vi "ControlMain.vi"() -> ()   [LabVIEW 2022 SP3]
panel:
  out "data out":string
  in  "stop":bool
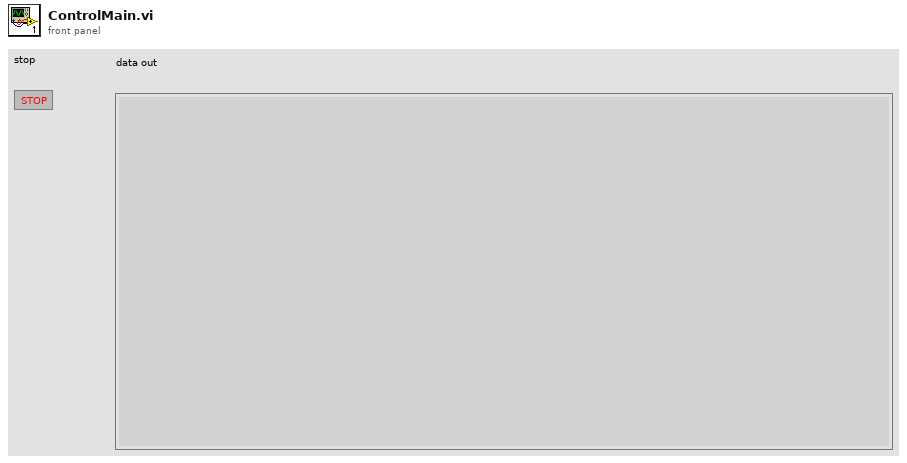
[diagram p1: front panel]
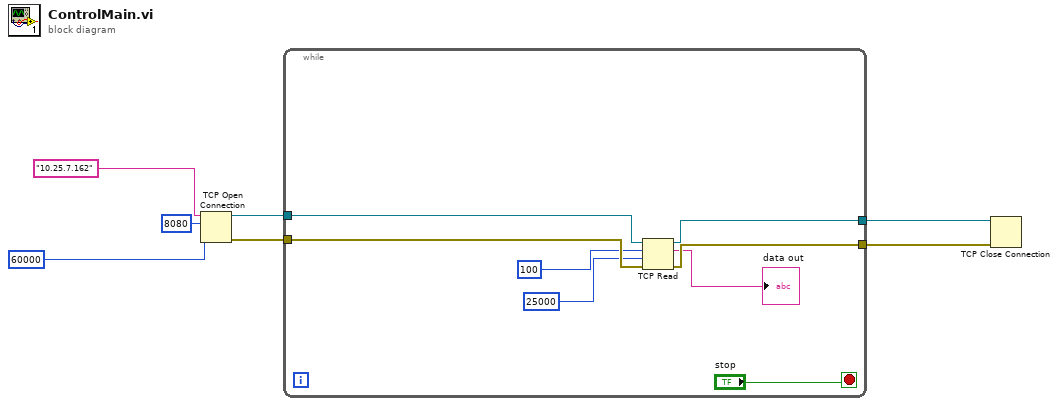
[diagram p0: block diagram]
diagram:
  n1 = TCP Open Connection(address="10.25.7.162", remote port or service name=u16 8080, timeout ms (60000)=60000) -> (connection ID=w3:refnum<k5>, error out=w4:errorcluster)  [unwired: 2 in]
  n2 = while {
    tunnel: w4 -> [w14]
    tunnel: w3 -> [w13]
    tunnel: [w12] -> w2
    tunnel: [w11] -> w1
    stop <- "stop" stop-if-true
    n3 = TCP Read(connection ID=w13, bytes to read=100, error in (no error)=w14, 9:25000 ("timeout ms (25000)")) -> (connection ID out=w11:refnum<k5>, data out=→"data out":string, error out=w12:errorcluster)  [unwired: 1 in]
  }
  n4 = TCP Close Connection(connection ID=w1, error in (no error)=w2) -> ()  [unwired: 1 in, 2 out]
